vi "do Logging.vi"(8 "error in (no error)":errorcluster, 10 "Content":string, 11 "File Logger in":refnum<class "File Logger.lvclass">) -> (0 "error out":errorcluster, 3 "File Logger out":refnum<class "File Logger.lvclass">)   [LabVIEW 2020, in "Logging.lvlib" / "File Logger.lvclass"]
uses:
  File Logger.lvclass
  File Logger.lvclass/File Logger.ctl
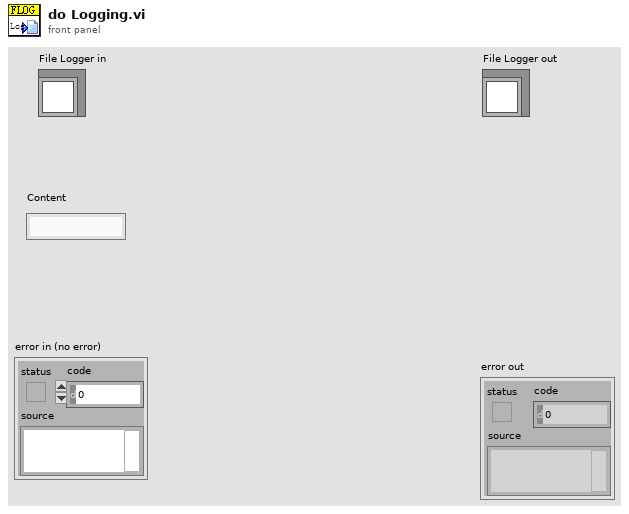
[diagram p1: front panel]
types:
  T1 = enum16{"open", "replace", "create", "open or create", "replace or create", "replace or create with confirmation"}
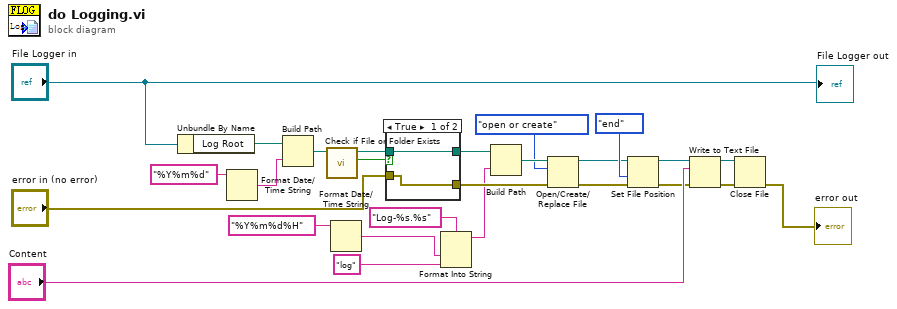
[diagram p0: block diagram]
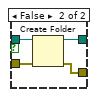
[diagram p2: hidden frame]
diagram:
  n1 = Unbundle By Name("File Logger in") -> ("Log Root"=w25:path)
  n2 = Format Date/Time String(time format string (%c)="%Y%m%d") -> (date/time string=w23:string)  [unwired: 2 in]
  n3 = Build Path(base path=w25, name or relative path=w23) -> (appended path=w22:path)
  n4 = call <vilib>:"Check if File or Folder Exists.vi"("path"=w22) -> ("file or folder exists?"=w21:bool, "dup path"=w20:path)  [unwired: 8 in, 1 out]
  n5 = Format Date/Time String(time format string (%c)="%Y%m%d%H") -> (date/time string=w10:string)  [unwired: 2 in]
  n6 = case shown="True" w21 {
    tunnel: w20 -> [w27 w32]
    tunnel: [w27 w31] -> w18
    tunnel: "error in (no error)" -> [w28 w30]
    tunnel: [w28 w29] -> w14
    frame True {
    }
    frame False {
      n7 = Create Folder(path (use dialog)=w32, error in=w30) -> (created path=w31:path, error out=w29:errorcluster)  [unwired: 1 in, 1 out]
    }
  }
  n8 = Format Into String(format string="Log-%s.%s", w10, "log" ("element")) -> (resulting string=w12:string)  [unwired: 2 in, 1 out]
  n9 = Build Path(base path=w18, name or relative path=w12) -> (appended path=w17:path)
  n10 = Open/Create/Replace File(file path (use dialog)=w17, error in=w14, operation (0:open)=T1."open or create") -> (refnum out=w4:refnum<file>, error out=w3:errorcluster)  [unwired: 3 in, 1 out]
  n11 = Set File Position(refnum=w4, from (0:start)=enum16{"start", "end", "current"}."end", error in=w3) -> (refnum out=w2:refnum<file>, error out=w1:errorcluster)  [unwired: 1 in]
  n12 = Write to Text File(file (use dialog)=w2, text="Content", error in=w1) -> (refnum out=w7:refnum<file>, error out=w6:errorcluster)  [unwired: 1 in, 1 out]
  n13 = Close File(refnum=w7, error in=w6) -> (error out=→"error out":errorcluster)  [unwired: 1 out]
  "File Logger out" <- "File Logger in"
